vi "DHE_CalcExptime.vi"(8 "error in (no error)":errorcluster, 10 "DHE_DBSRef":T1) -> (0 "error out":errorcluster, 1 "idle time":u32, 2 "total exp time":u32, 4 "min_exp_time":dbl)   [LabVIEW 2016]
uses:
  DBSHAND/private/vis/DatabaseHand_RefNum.ctl
  DBSHAND/private/vis/DatabaseHand_Element_Get(bool).vi
  DBSHAND/private/vis/DatabaseHand_Element_Get(double).vi
  DBSHAND/private/vis/DatabaseHand_Element_Set(double).vi
  DBSHAND/private/vis/DatabaseHand_Element_Get(I32).vi
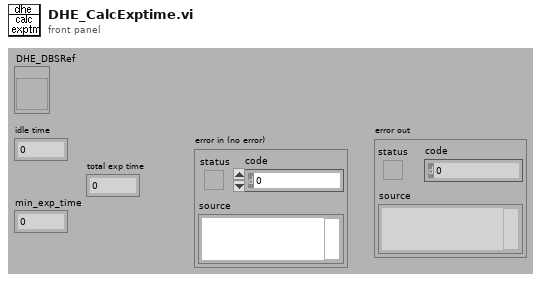
[diagram p1: front panel]
types:
  T1 = typedef "DatabaseHand_RefNum.ctl" = refnum<vi>
  T2 = cluster{"Video Processor Type":string, "support gain":bool, "Timing Board":string, "support reset":bool, "Utility Board":string, "Shutter":string, "Temperature":string, "support temp control":bool, "Detector Type":string, "Support MPP":string, "Support Binning":string, "Readout Mode":string, "support shutter control":bool}
  T3 = typedef "CMN_TimingInfo.ctl" = cluster{"PixelTime":sgl, "SkipPixel":sgl, "SkipRow":sgl, "ShiftRow":sgl, "ShiftedPix":u16, "known_overhead":sgl, "DET_READ_TIME":sgl}
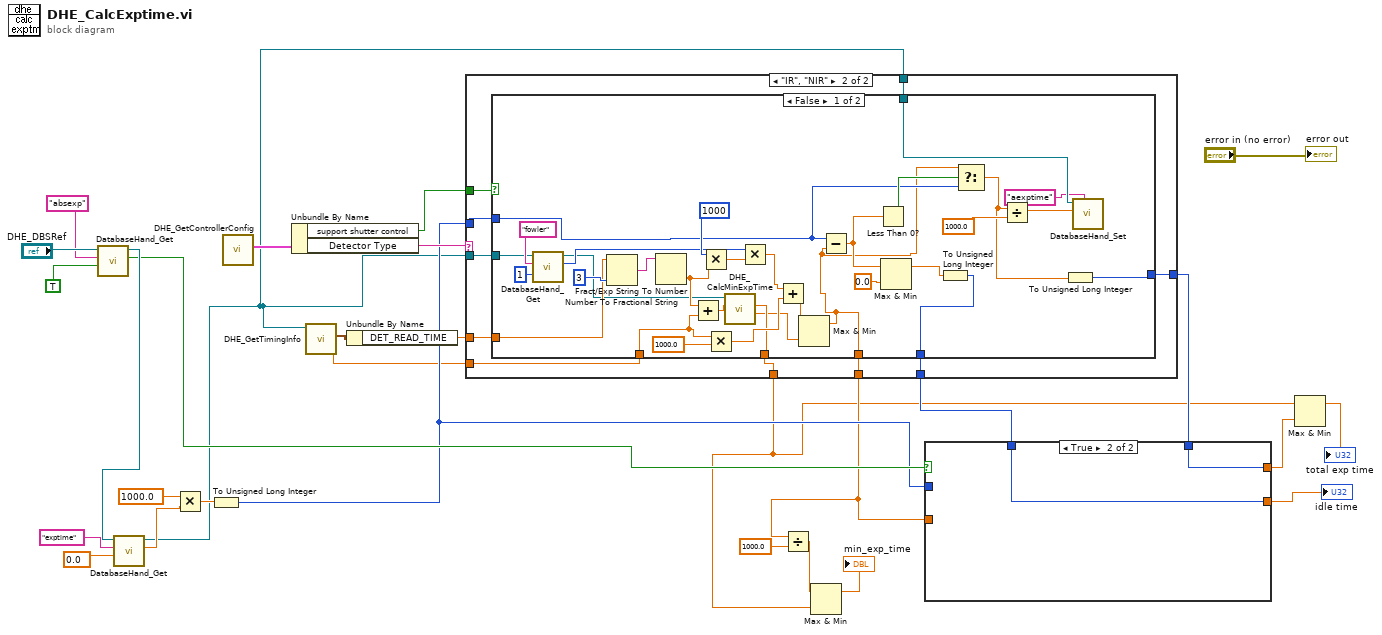
[diagram p0: block diagram]
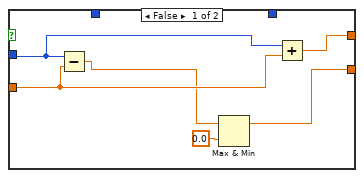
[diagram p2: hidden frame]
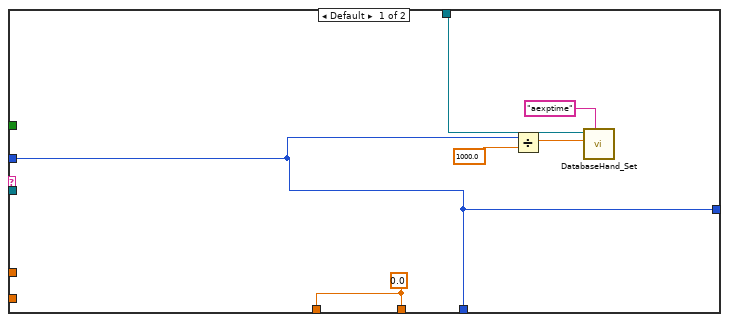
[diagram p3: hidden frame]
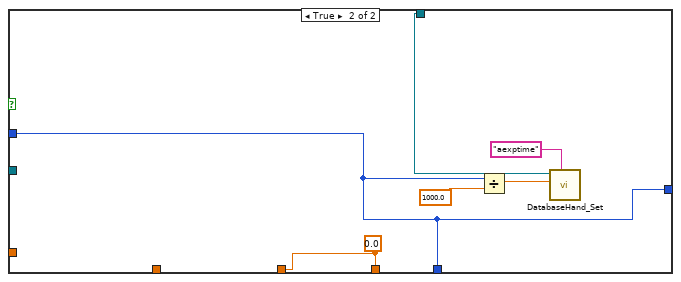
[diagram p4: hidden frame]
diagram:
  n1 = call-poly "DatabaseHand_Get.vi"("default value"=TRUE, "name"="absexp", "Database RefNum in"="DHE_DBSRef") -> ("value"=w17:bool, "Database RefNum out"=w21:T1)  [unwired: 2 in, 5 out]
  n2 = call-poly "DatabaseHand_Get.vi"("default value"=0.0, "name"="exptime", "Database RefNum in"=w21) -> ("value"=w24:dbl, "Database RefNum out"=w9:T1)  [unwired: 2 in, 5 out]
  n3 = Multiply(x=1000.0, y=w24) -> (x*y=w25:dbl)
  n4 = To Unsigned Long Integer(number=w25) -> (unsigned 32bit integer=w14:u32)
  n5 = call "DHE_GetControllerConfig.vi"() -> ("ControllerConfigCluster"=w20:T2)  [unwired: 11 out]
  n6 = Unbundle By Name(w20) -> ("support shutter control"=w4:bool, "Detector Type"=w19:string)
  n7 = call "DHE_GetTimingInfo.vi"("Database RefNum out"=w9) -> ("exposure_overhead"=w3:dbl, "Timing"=w10:T3)  [unwired: 9 out]
  n8 = Unbundle By Name(w10) -> ("DET_READ_TIME"=w18:sgl)
  n9 = case shown="\"IR\", \"NIR\"" w19 {
    tunnel: w14 -> [w33 w40]
    tunnel: [w33 w45] -> w16
    tunnel: w9 -> [_ w44]
    tunnel: [w33 w41] -> w13
    tunnel: w18 -> [_ w43]
    tunnel: w9 -> [w31 w42]
    tunnel: [w30 w39] -> w11
    tunnel: w4 -> [_ w38]
    tunnel: w3 -> [_ w37]
    tunnel: [w30 w36] -> w2
    frame Default {
      w30 = 0.0
      n10 = Divide(x=w33, y=1000.0) -> (x/y=w34:dbl)
      n11 = call-poly "DatabaseHand_Set.vi"("name"="aexptime", "value"=w34, "Database RefNum in"=w31) -> ()  [unwired: 5 in, 4 out]
    }
    frame "IR", "NIR" {
      n12 = case shown="False" w38 {
        tunnel: [w77 w79] -> w45
        tunnel: w44 -> [w70 _]
        tunnel: w43 -> [w65 _]
        tunnel: w42 -> [w64 w80]
        tunnel: [w63 w79] -> w41
        tunnel: w40 -> [w58 w79]
        tunnel: [w51 w78] -> w39
        tunnel: w37 -> [w49 _]
        tunnel: [w47 w78] -> w36
        frame False {
          n13 = call-poly "DatabaseHand_Get.vi"("default value"=1, "name"="fowler", "Database RefNum in"=w70) -> ("value"=w69:i32, "Database RefNum out"=w53:T1)  [unwired: 2 in, 5 out]
          n14 = Number To Fractional String(number=w65, precision (6)=i16 3) -> (F-format string=w75:string)  [unwired: 2 out]
          n15 = Fract/Exp String To Number(string=w75) -> (number=w55:dbl)  [unwired: 4 out]
          n16 = Add(x=w55, y=w49) -> (x+y=w54:dbl)
          n17 = Multiply(x=u32 1000 ("y"), y=w55) -> (x*y=w73:dbl)
          n18 = Multiply(x=w49, y=1000.0) -> (x*y=w48:dbl)
          n19 = call "DHE_CalcMinExpTime.vi"("calculated value in (s)"=w54, "Database RefNum out"=w53) -> ("min_exp_time(ms)"=w46:dbl, "min_exp_time(s)"=w47:dbl)  [unwired: 8 out]
          n20 = Multiply(x=w69, y=w73) -> (x*y=w56:dbl)
          n21 = Add(x=w56, y=w48) -> (x+y=w52:dbl)
          n22 = Max & Min(x=w52, y=w46) -> (max(x,y)=w51:dbl)  [unwired: 1 out]
          n23 = Subtract(x=w58, y=w51) -> (x-y=w68:dbl)
          n24 = Less Than 0?(x=w68) -> (x < 0?=w59:bool)
          n25 = Max & Min(x=w68, y=0.0) -> (max(x,y)=w66:dbl)  [unwired: 1 out]
          n26 = To Unsigned Long Integer(number=w66) -> (unsigned 32bit integer=w77:u32)
          n27 = Select(t=w51, s=w59, f=w58) -> (s? t:f=w57:dbl)
          n28 = Divide(x=w57, y=1000.0) -> (x/y=w60:dbl)
          n29 = To Unsigned Long Integer(number=w57) -> (unsigned 32bit integer=w63:u32)
          n30 = call-poly "DatabaseHand_Set.vi"("name"="aexptime", "value"=w60, "Database RefNum in"=w64) -> ()  [unwired: 5 in, 4 out]
        }
        frame True {
          w78 = 0.0
          n31 = Divide(x=w79, y=1000.0) -> (x/y=w82:dbl)
          n32 = call-poly "DatabaseHand_Set.vi"("name"="aexptime", "value"=w82, "Database RefNum in"=w80) -> ()  [unwired: 5 in, 4 out]
        }
      }
    }
  }
  n33 = Divide(x=w11, y=1000.0) -> (x/y=w8:dbl)
  n34 = Max & Min(x=w8, y=w2) -> (max(x,y)=→"min_exp_time":dbl)  [unwired: 1 out]
  n35 = case shown="True" w17 {
    tunnel: w16 -> [_ w91]
    tunnel: [w84 w91] -> w15
    tunnel: w14 -> [w88 _]
    tunnel: w11 -> [w89 _]
    tunnel: w13 -> [_ w90]
    tunnel: [w87 w90] -> w5
    frame False {
      n36 = Subtract(x=w88, y=w89) -> (x-y=w85:dbl)
      n37 = Max & Min(x=w85, y=0.0) -> (max(x,y)=w84:dbl)  [unwired: 1 out]
      n38 = Add(x=w88, y=w89) -> (x+y=w87:dbl)
    }
    frame True {
    }
  }
  "idle time" <- w15
  n39 = Max & Min(x=w2, y=w5) -> (max(x,y)=→"total exp time":dbl)  [unwired: 1 out]
  "error out" <- "error in (no error)"
